vi "FGV_OBJ_history_display.vi"(4 "front_panel_reference":refnum<vi>, 6 "history_display_reference":refnum<vi>, 7 "options":T1, 8 "error_in":errorcluster, 11 "input":variant) -> (0 "error_out":errorcluster)   [LabVIEW 2019]
uses:
  FGV_OBJ_history_display.ctl
  OBJ_records_display/OBJ_all_info.ctl
  MAIN/OBJ_header_data_display.ctl
  MAIN/OBJ_measurement_status.ctl
  OBJ_records_display/OBJ_references.ctl
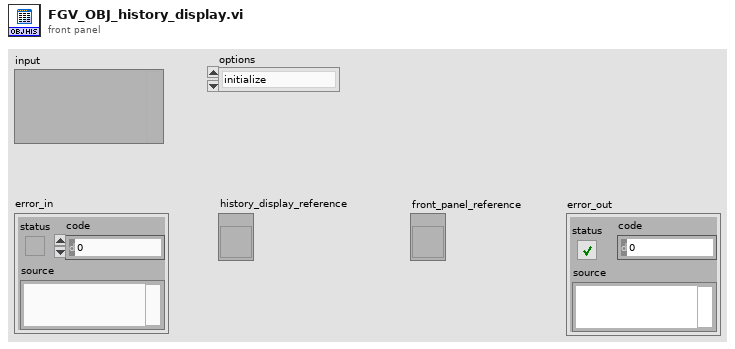
[diagram p1: front panel]
types:
  T1 = typedef "FGV_OBJ_history_display.ctl" = enum16{"initialize", "add", "clear"}
  T2 = typedef "OBJ_all_info.ctl" = cluster{"serial":string, "OBJ_header":T3, "ItemNames":string[][], "statuses":T4[], "OBJ_references":T5}
  T3 = typedef "OBJ_header_data_display.ctl" = cluster{"ID":string, "creation_time":string, "last_station":string, "last_status":string, "pinion_serial":string, "batch_code":string}
  T4 = typedef "OBJ_measurement_status.ctl" = enum16{"OK", "NOK"}
  T5 = typedef "OBJ_references.ctl" = cluster{"front_panel_reference":refnum<vi>, "SQL_listbox_reference":refnum<vi>, "OBJ_header_data_display":refnum<vi>}
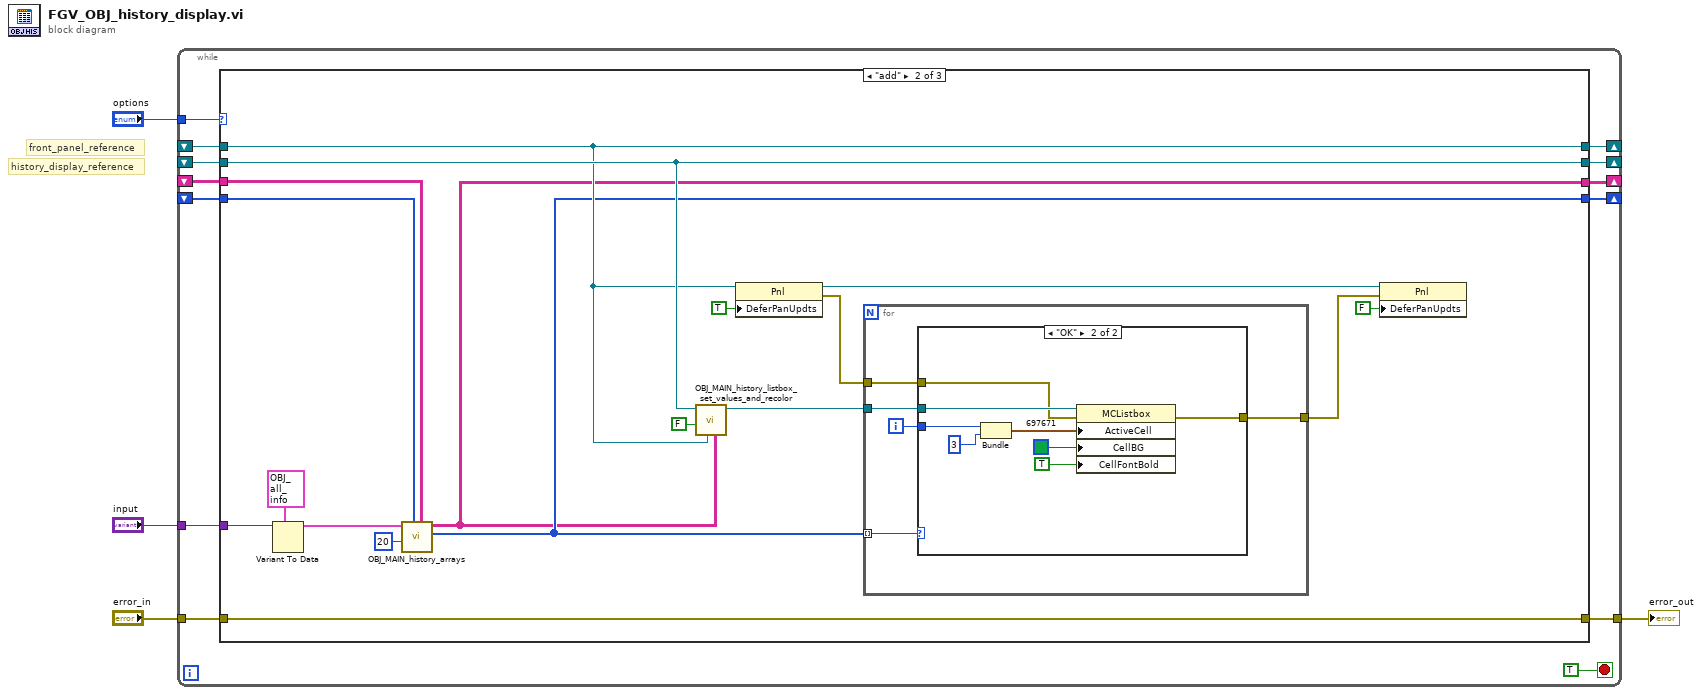
[diagram p0: block diagram]
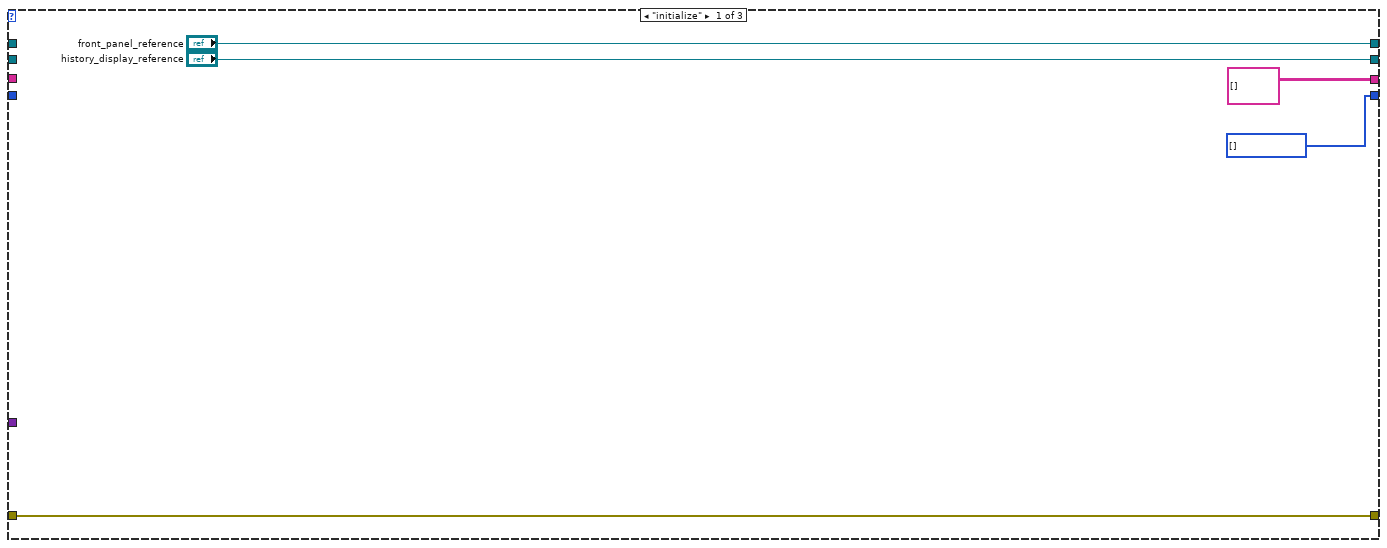
[diagram p2: hidden frame]
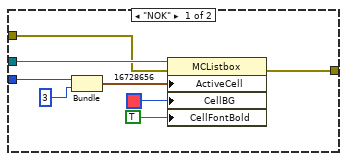
[diagram p3: hidden frame]
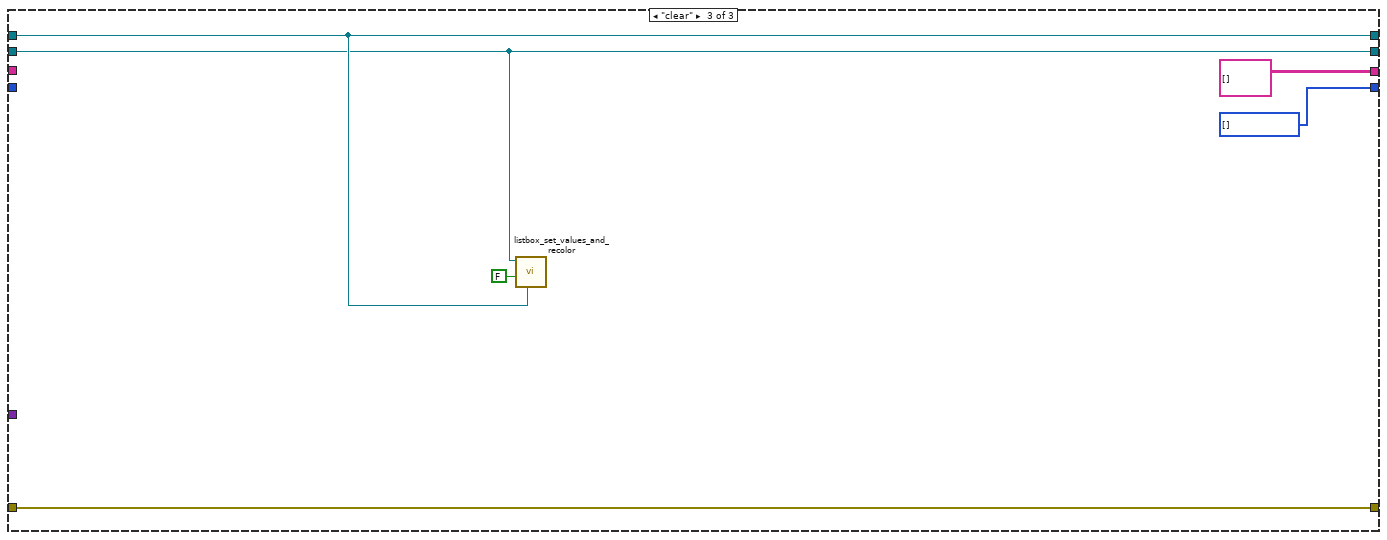
[diagram p4: hidden frame]
diagram:
  # "history_display_reference"
  # "front_panel_reference"
  n1 = while {
    tunnel: "options" -> [w16]
    tunnel: [w15] -> w4
    tunnel: "error_in" -> [w14]
    tunnel: "input" -> [w13]
    shift-right: [w12] -> _
    shift-left: _ -> [w10]
    shift-right: [w11] -> _
    shift-left: _ -> [w9]
    shift-right: [w8] -> _
    shift-left: _ -> [w6]
    shift-right: [w7] -> _
    shift-left: _ -> [w5]
    stop <- TRUE stop-if-true
    n2 = case shown="\"add\"" w16 {
      tunnel: [w22 w40 w67] -> w15
      tunnel: w14 -> [w22 w40 w67]
      tunnel: w13 -> [_ w39 _]
      tunnel: ["front_panel_reference" w29 w65] -> w12
      tunnel: ["history_display_reference" w32 w64] -> w11
      tunnel: w10 -> [_ w29 w65]
      tunnel: w9 -> [_ w32 w64]
      tunnel: [string[][] [] ("item_names_out") w24 string[][] [] ("item_names_out")] -> w8
      tunnel: [w18 w27 w62] -> w7
      tunnel: w6 -> [_ w25 _]
      tunnel: w5 -> [_ w26 _]
      frame "initialize" {
        w18 = T4[] [] items=["OK", "NOK"] ("statuses_out")
      }
      frame "add" {
        n3 = Variant To Data(type=T2 {"serial"="", "OBJ_header"={"ID"="", "creation_time"="", "last_station"="", "last_status"="", "pinion_serial"="", "batch_code"=""}, "ItemNames"=[], "statuses"=[], "OBJ_references"={"front_panel_reference"=refnum, "SQL_listbox_reference"=refnum, "OBJ_header_data_display"=refnum}} ("output cluster"), Variant=w39) -> (data=w28:T2)  [unwired: 1 in, 1 out]
        n4 = call "OBJ_MAIN_history_arrays.vi"("item_names_in"=w25, "statuses_in"=w26, "tests_to_remember"=20, "output cluster"=w28) -> ("statuses_out"=w27:T4[], "item_names_out"=w24:string[][])  [unwired: 6 in]
        n5 = call "OBJ_MAIN_history_listbox_set_values_and_recolor.vi"("item_names"=w24, "front_panel_reference"=w29, "Autosize? (T)"=FALSE, "multicolumn_listbox_reference_in"=w32) -> ("multicolumn_listbox_reference_out"=w31:refnum<vi>)  [unwired: 6 in, 1 out]
        n6 = property class="Pnl"(reference=w29, "DeferPanUpdts"=TRUE ("Defer Panel Updates")) -> (reference out=w35:refnum<vi>, error out=w33:errorcluster)  [unwired: 1 in]
        n7 = for {
          tunnel: w31 -> [w45]
          tunnel: w27 -> [w44] mode=indexing
          tunnel: [w42] -> w34
          tunnel: w33 -> [w41]
          i -> [w43]
          n8 = case shown="\"OK\"" w44 {
            tunnel: w45 -> [w51 w60]
            tunnel: w43 -> [w50 w59]
            tunnel: [w47 w54] -> w42
            tunnel: w41 -> [w46 w55]
            frame "NOK" {
              n9 = Bundle(w50, 3) -> (w52:cluster{i32, i32})  [unwired: 1 in]
              n10 = property on="Property Node" class="MCListbox"(reference=w51, error in=w46, "ActiveCell"=w52, "CellBG"=u32 16728656, "CellFontBold"=TRUE ("Active Cell:Cell Font:Bold")) -> (error out=w47:errorcluster)  [unwired: 1 out]
            }
            frame "OK" {
              n11 = Bundle(w59, 3) -> (w57:cluster{i32, i32})  [unwired: 1 in]
              n12 = property on="Property Node" class="MCListbox"(reference=w60, error in=w55, "ActiveCell"=w57, "CellBG"=u32 697671, "CellFontBold"=TRUE ("Active Cell:Cell Font:Bold")) -> (error out=w54:errorcluster)  [unwired: 1 out]
            }
          }
        }
        n13 = property class="Pnl"(reference=w35, error in=w34, "DeferPanUpdts"=FALSE ("Defer Panel Updates")) -> ()  [unwired: 2 out]
      }
      frame "clear" {
        w62 = T4[] [] items=["OK", "NOK"] ("statuses_out")
        n14 = call "listbox_set_values_and_recolor.vi"("front_panel_reference"=w65, "Autosize? (T)"=FALSE, "multicolumn_listbox_reference_in"=w64) -> ()  [unwired: 7 in, 2 out]
      }
    }
  }
  "error_out" <- w4
